vi "VI Erw. Konfig.vi"() -> ()   [LabVIEW 2020, in "Erweiterte Konfig.lvlib"]
uses:
  Seiten/Erweiterte Konfig/Erweiterte Konfig.lvlib
  Seiten/Erweiterte Konfig/PID-Parameter Anzeige.ctl
  Seiten/Erweiterte Konfig/PID-Parameter.ctl
  Visualisierungs Elemente/Zahlen-Eingabefeld.ctl
  Visualisierungs Elemente/Zahlen-Ausgabefeld.ctl
  Visualisierungs Elemente/Button.ctl
  Visualisierungs Elemente/Auswahlfeld.ctl
  Seiten/Erweiterte Konfig/Dichtheitstest Umfang.ctl
  Seiten/Erweiterte Konfig/Cluster LN2 normal.ctl
  Seiten/Erweiterte Konfig/Ventilanzeige.ctl
  Seiten/Erweiterte Konfig/Cluster Extern LN2.ctl
  Visualisierungs Elemente/String - Ausgabefeld.ctl
  Seiten/Erweiterte Konfig/Parameter Sensoren.ctl
  Seiten/Erweiterte Konfig/Aktionen Stickstoff Befuellung.ctl
  Seiten/Erweiterte Konfig/Aktionen Externe Stockstoff Befuellung.ctl
  Seiten/Erweiterte Konfig/FGV PID Aktionen.ctl
  Seiten/Log Konfig/Auswahlfeld aktiviert-deaktiviert.ctl
  Sprachverwaltung/FGV Aktion Tabelle zerlegen.ctl
  Passwortverwaltung/FGV Passwort Aktion.ctl
  Allgemein/Aktionen Daten am cRIO speichern.ctl
  Funktionstasten/Funktionstasten-Aktion.ctl
  Funktionstasten/Zustaende.ctl
  T90/T90 konfig.vi
  Seiten/Erweiterte Konfig/Parameter Druck Sensoren.vi
  Seiten/Erweiterte Konfig/PID-Parameter Druckregler einstellen v2.vi
  AK-Schnittstelle/Konfig AK.vi
  O2 Dichtheitstest/O2 main.vi
  Seiten/Erweiterte Konfig/Konfig CG-Check/VI CG-Check Konfig.vi
  Passwortverwaltung/Passwort.lvlib
  cRIO/PC/Kommunikation mit cRIO.lvlib
  Allgemein/allgemeine Sub-VIs.lvlib
  Funktionstasten/Funktionstasten.lvlib
  AK-Schnittstelle/AK-Schnittstelle.lvlib
  Seiten/Log Konfig/LogKonfig.lvlib
  T90/T90.lvlib
  Seiten/Erweiterte Konfig/Konfig CG-Check/CG-Check Konfig.lvlib
  O2 Dichtheitstest/O2 Dichtheitstest.lvlib
  Sprachverwaltung/Sprachverwaltung.lvlib
panel:
  in  "Aktion Externe Stickstoffbefüllung":T1
  in  "Aktion Stick":T2
  in  "O2 Dichtheitstest":T3 caption="Dichtheitstest"
  in  "Pumpendrehzahl":sgl=50.0 caption="Pumpendrehzahl:" min=50 max=100 format="%#_5g"
  in  "CG-Konfig":T3 caption="Dichtheitstest"
  out "Taupunkt":T4 caption="°C" format="%.1f"
  in  "Max Taupunkt":T5 caption="Offset Ausgang" format="%.1f"
  in  "Sensor Parameter":T3 caption="Status Digital IO"
  in  "Manueller Betrieb":bool
  in  "Gasringverdichter Speed":dbl(knob) scale=0.0..5.0
  out "Druck Umgebung:":T4 caption="mbar"
  in  "Offset Umgebung":T5 format="%#_5g"
  out "Rohwert Umgebung":T4 format="%.3f"
  out "Druck Ausgang:":T4 caption="mbar"
  in  "Offset Ausgang":T5 format="%#_5g"
  out "Rohwert Ausgang":T4 format="%.3f"
  in  "speichern":T3
  in  "T90":T3
  in  "Dichtheitstest":T3
  in  "Parameter Druckregler":T3
  in  "Status Digital IO":T3
  in  "Config AK":T3
  out "Klima Einschalten":string
  out "Klima":string
  in  "Schnell ab:":T5 caption="°C" format="%#_5g"
  in  "Lüfter langsam":T5 format="%#_5g"
  out "Rohwert Druck FT-IR":T4 format="%.3f"
  in  "Offset Druck FT-IR":T5 format="%#_5g"
  out "FT-IR Druck Ist":T4 format="%.3f"
  in  "Offset FT-IR":T5 format="%#_5g"
  out "Rohwert FT-IR":T4 format="%.3f"
  in  "Kalib.FT-IR":T5 format="%#_5g"
  in  "Registerkartenelement":T6(tab)
  in  "Dichtheitstest Umfang":T7 items=["FT-IR/PNS/HL to LeakValve", "FT-IR/PNS"]
  in  "Überwachung":T8 items=["Normaler Betrieb mit Überwachung", "Überwachung deaktiviert (TESTBETRIEB!!!!)"]
  in  "FT-IR Kühlung Max":T5 format="%.1f"
  out "FT-IR Kühlung Ist":T4 format="%.1f"
  in  "Dichtheitstest Zeit":T5 format="%#_5g"
  in  "Dichtheitstest Abfall":T5 format="%#_5g"
  in  "°C":T5 caption="Sollwert:" format="%.1f"
  in  "LN2 Cluster mit Ext":T9 {"Stickstoff Befüllzeit Ext" format="%#_5g"; "Befüllintervall" format="%#_5g"; "Stickstoff Befüllzeit" format="%#_5g"; "Befüllung Extern aktiv" items=["Deaktiviert", "Aktiviert"]; "Befüllung aktiv" items=["Deaktiviert", "Aktiviert"]}
  in  "LN2 normal":T12 {"Befüllung aktiv" items=["Deaktiviert", "Aktiviert"]; "Befüllintervall" format="%#_5g"; "Stickstoff Befüllzeit" format="%#_5g"}
  out "PMA unsichtbar schalten":bool
  out "Roh Druck Kalter Block":sgl caption="V" format="%.3f"
  out "Druck Kalter Block":sgl caption="bar" format="%.2f"
  out "Roh Durck FTIR IAG":sgl caption="V" format="%.3f"
  out "Roh Durck CG":sgl caption="V" format="%.3f"
  out "Roh Druck CG PMA":sgl caption="V" format="%.3f"
  out "Roh Durchfl.PMA":sgl caption="V" format="%.3f"
  out "Roh Durck Umgebung":sgl caption="V" format="%.3f"
  out "Roh Druck Ausgang":sgl caption="V" format="%.3f"
  out "Roh Durchfl.FTIR":sgl caption="V" format="%.3f"
  out "Druck FTIR IAG":sgl caption="atm" format="%.3f"
  out "Druck CG":sgl caption="bar" format="%.2f"
  out "Druck CG PMA":sgl caption="bar" format="%.2f"
  out "Druck Umgebung":sgl caption="mbar" format="%#.0f"
  out "Druck Ausgang":sgl caption="mbar" format="%#.0f"
  out "Durchfluss PMA":sgl caption="l/min" format="%.1f"
  out "Durchfluss FTIR":sgl caption="l/min" format="%.1f"
  in  "Parameter Sensoren":T13 {"Druck Kalter Block" format="%#_5g"; "Offset Druck FTIR IAG" format="%#_5g"; "Offset Druck CG" format="%#_5g"; "Offset Druck CG PMA" format="%#_5g"; "Offset Durchfl.PMA" format="%#_5g"; "Offset Druck Umgebung" format="%#_5g"; "Offset Druck Ausgang" format="%#_5g"; "Offset Durchfl.FTIR" format="%#_5g"; "Kal.Durchfl.PMA" format="%.3g"; "Kal.Durchfl.FTIR" format="%.3g"}
  in  "PID-Parameter Anzeige":T14 {"Heizung\nHeizleitungen"."max. OUT" format="%#_5g"; "Heizung\nHeizleitungen"."Regelzonengr." format="%#_5g"; "Heizung\nHeizleitungen"."D-Anteil" format="%#_5g"; "Heizung\nHeizleitungen"."I-Anteil" format="%#_5g"; "Heizung\nHeizleitungen"."P-Anteil" format="%.1f"; "Heizleitung\nExtern"."max. OUT" format="%#_5g"; "Heizleitung\nExtern"."Regelzonengr." format="%#_5g"; "Heizleitung\nExtern"."D-Anteil" format="%#_5g"; "Heizleitung\nExtern"."I-Anteil" format="%#_5g"; "Heizleitung\nExtern"."P-Anteil" format="%.1f"; "Heizung\nFB-Druckregler"."max. OUT" format="%#_5g"; "Heizung\nFB-Druckregler"."Regelzonengr." format="%#_5g"; "Heizung\nFB-Druckregler"."D-Anteil" format="%#_5g"; "Heizung\nFB-Druckregler"."I-Anteil" format="%#_5g"; "Heizung\nFB-Druckregler"."P-Anteil" format="%.1f"; "Heizung\nPumpe"."max. OUT" format="%#_5g"; "Heizung\nPumpe"."Regelzonengr." format="%#_5g"; "Heizung\nPumpe"."D-Anteil" format="%#_5g"; "Heizung\nPumpe"."I-Anteil" format="%#_5g"; "Heizung\nPumpe"."P-Anteil" format="%.1f"; "Heizung\nFilterblock"."max. OUT" format="%#_5g"; "Heizung\nFilterblock"."Regelzonengr." format="%#_5g"; "Heizung\nFilterblock"."D-Anteil" format="%#_5g"; "Heizung\nFilterblock"."I-Anteil" format="%#_5g"; "Heizung\nFilterblock"."P-Anteil" format="%.1f"}
  # "Erweiterte Konfig"
  # "°C"
  # "%"
  # "Taupunktsensor:"
  # "Istwert:"
  # "°C"
  # "Max. Wert:"
  # "Istwert:"
  # "Umgebungsdruck:"
  # "Offset:"
  # "mbar"
  # "Rohwert:"
  # "V"
  # "Istwert:"
  # "Druck Ausgang:"
  # "Offset:"
  # "mbar"
  # "Rohwert:"
  # "V"
  # "Istwert:"
  # "Druck FT-IR IAG:"
  # "atm"
  # "Offset:"
  # "atm"
  # "Rohwert:"
  # "V"
  # "Durchfluss FT-IR:"
  # "Kalibrierwert:"
  # "Offset:"
  # "Rohwert:"
  # "V"
  # "Dichtheitstest:"
  # "max. Druckanstieg:"
  # "mbar"
  # "Kühlung FT-IR:"
  # "Max. Wert:"
  # "°C"
  # "Überwachung von Grundbedingnungen:"
  # "Istwert:"
  # "°C"
  # "Prüfzeit:"
  # "sec"
  # "Parameter interne Flüssig-Stickstoff-Nachfüllung"
  # "Parameter externe Flüssig-Stickstoff-Nachfüllung"
  # "PA"
  # "3"
  # "Externer\nDewar 50l"
  # "Dewar 4l"
  # "FT-IR"
  # "Zeitdauer letzter Füllvorgang:"
  # "sec"
  # "Fülldauer wenn Sensor erkannt:"
  # "sec"
  # "Befüllintervall:"
  # "Stunden"
  # "Zeitdauer letzter Füllvorgang:"
  # "sec"
  # "Fülldauer wenn Sensor erkannt:"
  # "sec"
  # "N2"
  # "5"
  # "CA"
  # "3"
  # "LS"
  # "-16B1"
  # "LS"
  # "-17B2"
  # "LS"
  # "-16B2"
  # "LS"
  # "-17B3"
  # "PR"
  # "0,2bar"
  # "Parameter interne Flüssig-Stickstoff-Nachfüllung"
  # "Zustand Befüllsystem:"
  # "Befüllintervall:"
  # "Stunden"
  # "Zeitstempel - letzter Füllvorgang:"
  # "Zeitdauer letzter Füllvorgang:"
  # "sec"
  # "Fülldauer wenn Sensor erkannt:"
  # "sec"
  # "Zeitstempel - vorletzter Füllvorgang:"
  # "Dewar 4l"
  # "FT-IR"
  # "N2"
  # "5"
  # "CA"
  # "3"
  # "LS"
  # "-16B1"
  # "LS"
  # "-16B2"
  # "Sensor"
  # "Istwert"
  # "Kalibrierwert"
  # "Offset"
  # "Rohwert"
  # "Durchfluss FT-IR:"
  # "Druck Ausgang:"
  # "Ambient Pressure:"
  # "Druck Calgas:"
  # "Druck FT-IR IAG:"
  # "Fluss PMA:"
  # "Druck CG PMA:"
  # "Druck Kalter Block:"
  # "PID -Parameter:"
  # "Verstärkung KR:"
  # "Nachstellzeit TN:"
  # "Vorhaltezeit TD:"
  # "Regelzonengrenze:"
  # "max. Ausgang:"
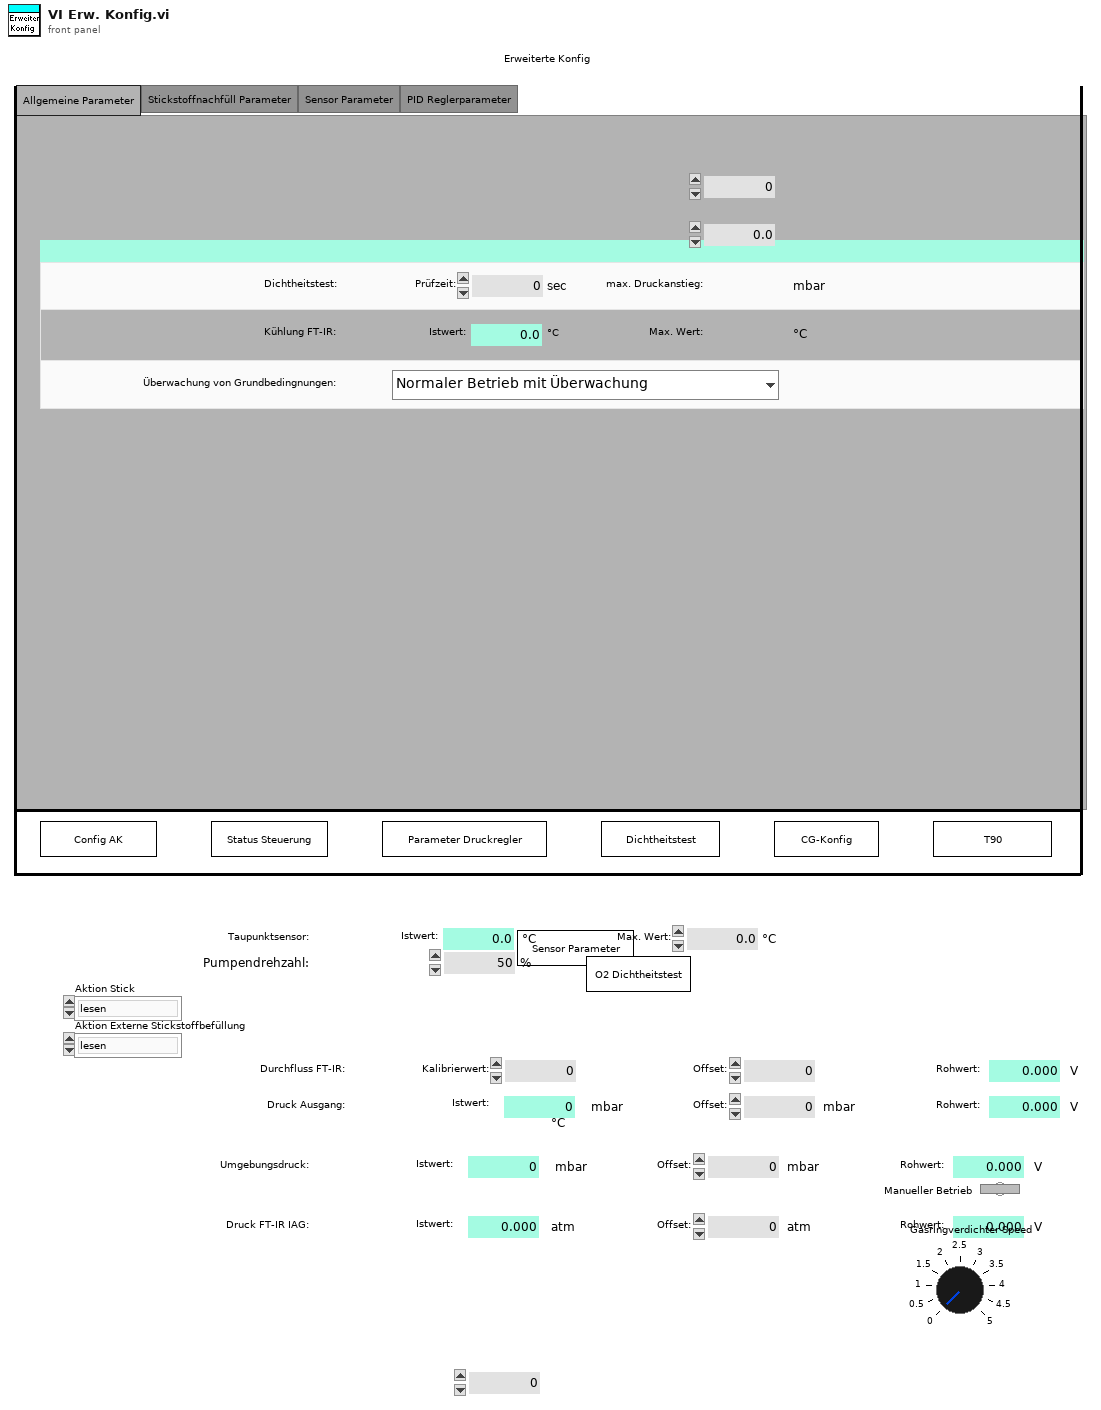
[diagram p1: front panel]
types:
  T1 = typedef "Erweiterte Konfig.lvlib/Aktionen Externe Stockstoff Befuellung.ctl" = enum16{"lesen", "Befüllen vorbereiten", "Befüllen", "Befüllen beenden", "Warten", "deaktiviert", "initialisieren"}
  T2 = typedef "Erweiterte Konfig.lvlib/Aktionen Stickstoff Befuellung.ctl" = enum16{"lesen", "Befüllen vorbereiten", "Befüllen", "Befüllen beenden", "Warten", "deaktiviert", "initialisieren"}
  T3 = typedef "Button.ctl" = bool
  T4 = typedef "Zahlen-Ausgabefeld.ctl" = sgl
  T5 = typedef "Zahlen-Eingabefeld.ctl" = sgl
  T6 = enum32{"General Parameters", "Liquid Nitrogen Parameters", "Sensor Parameter", "PID Regulate Parameters"}
  T7 = typedef "Erweiterte Konfig.lvlib/Dichtheitstest Umfang.ctl" = u16
  T8 = typedef "Auswahlfeld.ctl" = u16
  T9 = typedef "Erweiterte Konfig.lvlib/Cluster Extern LN2.ctl" = cluster{"Befüllung aktiv":u16, "Zeitstempel":timestamp, "Zeitstempel 2":timestamp, "Status LN2 Befüllung":T10, "Befüllintervall":T5, "Zeit Füllvorgang":T4, "Stickstoff Befüllzeit":T5, "Befüllung Extern aktiv":u16, "Zeitstempel 1 Ext":timestamp, "Zeitstempel 2 Ext":timestamp, "Status LN2 Befüllung Ext.":T10, "Zeit Füllvorgang Ext":T4, "Stickstoff Befüllzeit Ext":T5, "LS -17B3":bool, "LS -16B2":bool, "LS -17B2":bool, "-22Y3 ":T11, "-22Y1":T11, "LS -16B1":bool, "-16B7":bool, "-22Y2":T11}
  T10 = typedef "String - Ausgabefeld.ctl" = string
  T11 = typedef "Erweiterte Konfig.lvlib/Ventilanzeige.ctl" = bool
  T12 = typedef "Erweiterte Konfig.lvlib/Cluster LN2 normal.ctl" = cluster{"Zeitstempel":timestamp, "Zeitstempel 2":timestamp, "Zeit Füllvorgang":T4, "Stickstoff Befüllzeit":T5, "Befüllintervall":T5, "Befüllung aktiv":u16, "-22Y1":T11, "-22Y2":T11, "LS -16B1":bool, "LS -16B2":bool}
  T13 = typedef "Erweiterte Konfig.lvlib/Parameter Sensoren.ctl" = cluster{"Kal.Durchfl.FTIR":sgl, "Kal.Durchfl.PMA":sgl, "Offset Durchfl.FTIR":sgl, "Offset Druck Ausgang":sgl, "Offset Druck Umgebung":sgl, "Offset Durchfl.PMA":sgl, "Offset Druck CG PMA":sgl, "Offset Druck CG":sgl, "Offset Druck FTIR IAG":sgl, "Druck Kalter Block":sgl}
  T14 = typedef "Erweiterte Konfig.lvlib/PID-Parameter Anzeige.ctl" = cluster{"Heizung\nFilterblock":T15, "Heizung\nPumpe":T15, "Heizung\nHeizleitungen":T15, "Heizleitung\nExtern":T15, "Heizung\nFB-Druckregler":T15}
  T15 = typedef "Erweiterte Konfig.lvlib/PID-Parameter.ctl" = cluster{"P-Anteil":T5, "I-Anteil":T5, "D-Anteil":T5, "Regelzonengr.":T5, "max. OUT":T5}
  T16 = typedef "Sprachverwaltung.lvlib/FGV Aktion Tabelle zerlegen.ctl" = enum16{"laden", "vereinzeln", "speichern"}
  T17 = enum8{"Enabled", "Disabled", "Disabled and Grayed Out"}
  T18 = typedef "Erweiterte Konfig.lvlib/FGV PID Aktionen.ctl" = enum16{"Lesen", "Schreiben PID", "Schreiben Sonstige", "Dichtheitstest", "Aktionen Dicht.", "Parameter Sensor"}
  T19 = typedef "LogKonfig.lvlib/Auswahlfeld aktiviert-deaktiviert.ctl" = u16
  T20 = typedef "Erweiterte Konfig.lvlib/Sonstige Parameter.ctl" = cluster{"Lüfter langsam":sgl, "Lüfter schnell":sgl, "FT-IR Kühlung Soll":sgl, "FT-IR Kühlung Max":sgl, "Überwachung":T8, "Befüllung aktiv":T19, "Stickstoff Befüllzeit":sgl, "Befüllintervall":sgl, "Kalibrierwert FT-IR":sgl, "Offset Ausgang":sgl, "Offset FT-IR":sgl, "Offset Druck FT-IR":sgl, "Dichtheitstest Zeit":sgl, "Dichtheitstest Abfall":sgl, "Dichtheitstest Umfang":T7, "Offset Umgebung":sgl, "Max Taupunkt":sgl, "Pumpendrehzahl":sgl, "ext. Befüllung":T19, "Ext. Stickstoff Befüllzeit":sgl}
  T21 = typedef "Passwort.lvlib/FGV Passwort Aktion.ctl" = enum16{"prüfen", "setzen", "Initialisieren", "PW speichern", "lesen", "PW Änderung"}
  T22 = typedef "allgemeine Sub-VIs.lvlib/Aktionen Daten am cRIO speichern.ctl" = enum16{"lesen", "speichern setzen", "speichern reset", "gespeichert"}
  T23 = typedef "Funktionstasten.lvlib/Zustaende.ctl" = enum16{"Standby", "Pause", "Eco", "Messen", "Kalibrieren", "Spülen Filter", "Spülen Leitung", "Umgebungsluft", "0-Gas", "Cal-Gas", "CG zu PNS", "-------------", "Init 1", "Init 2", "Init 3", "Init 4", "Messen vorbereiten", "Messen durchführen", "Exit"}
  T24 = typedef "Funktionstasten.lvlib/Funktionstasten-Aktion.ctl" = enum16{"Initialisieren", "Zustand setzen", "Taste gedrückt", "Fehler speichern", "Lesen", "Manuell", "Remote", "Bitparallel", "Samplepoint", "Zeit Prüfen", "reset Umschalten"}
  T25 = typedef "Verwaltung - cRIO.lvlib/Digital Eingaenge 0-15.ctl" = cluster{"I0: N2 Nachf. FT-IR voll":bool, "I1: N2 Nachf. Vorrat leer":bool, "I2: (Klimaanlage eingeschaltet)":bool, "I3: (Klimaanlage Störung)":bool, "I4: Trigger Eingang (Messdaten sp.)":bool, "I5: Reserve":bool, "I6: Reserve":bool, "I7: Reserve":bool, "I8: Druckschalter Versorgung ok":bool, "I9: Reserve":bool, "I10: Reserve":bool, "I11: Reserve":bool, "I12: Drucksch. N2 Versorgung":bool, "I13: Reserve":bool, "I14: Drucksch. N2 Optikbox":bool, "I15: (Füllstand Kondensatbehälter)":bool}
  T26 = typedef "Verwaltung - cRIO.lvlib/Digital Ausgaenge 0-31.ctl" = cluster{"O0: Druckluft Versorgung":bool, "O1: CG 1 (FB Eingang 1)":bool, "O2: CG 2 (Kühlung FT-IR EIN)":bool, "O3: CG 3 (FB Bypass)":bool, "O4: CG 4 (FB CalGas)":bool, "O5: CG 5 (FB spülen/UL)":bool, "O6: CG 6 (FB zum FT-IR)":bool, "O7: CG 7 (FB zum FID)":bool, "O8: CG 8 (FB Reserve)":bool, "O9: (FB Reserve)":bool, "O10: (FB Umgebungsluft FID)":bool, "O11: (FB zum Gaskühler)":bool, "O12: FB Stickstoff zu FT-IR":bool, "O13: Optikbox FT-IR spülen":bool, "O14: (Purifier deaktivieren)":bool, "O15: (Umschaltung Purifier/Stickstoff)":bool, "O16: N2 Einblasung":bool, "O17: LSP LN2 Nachfüllung":bool, "O18: (Reserve)":bool, "O19: (Pumpe Eingang1)":bool, "O20: (Pumpe Eingang2)":bool, "O21: (Pumpe Spülen1)":bool, "O22: (Pumpe Spülen2)":bool, "O23: (Reserve)":bool, "O24: CalGas 1":bool, "O25: CalGas 2":bool, "O26: CG 3-8 (CalGas 3)":bool, "O27: Stickstoff aufschalten":bool, "O28: CG zu PNS":bool, "O29: FTIR Standby Spülung":bool, "O30: CG zu Entnahme(T90)":bool, "O31: (Purifier regenerieren)":bool}
  T27 = typedef "Verwaltung - cRIO.lvlib/Digital Ausgaenge 32-63.ctl" = cluster{"O32: Messgaspumpe EIN":bool, "O33: (Umgebungsluftpumpe)":bool, "O34: (Kondensatpumpe GK)":bool, "O35: Klima/Lüfter EIN":bool, "O36: Versorgung Heizungen":bool, "O37: Versorgung Heizungen":bool, "O38: (Gaskühler EIN (Freigabe))":bool, "O39: Störung FAS LP":bool, "O40: (Heizung Filterblock)":bool, "O41: Heizung HL zu FT-IR":bool, "O42: Heizung HL Extern SP1":bool, "O43: Heizung HL Extern SP2":bool, "O44: Heizung Reserve":bool, "O45: Heizung Reserve":bool, "O46: Statusbeleuchtung grün":bool, "O47: Statusbeleuchtung rot":bool}
  T28 = typedef "Verwaltung - cRIO.lvlib/Analog Eingaenge.ctl" = cluster{"AI0: Durchfluss FT-IR":sgl, "AI1: Druck Ausgang":sgl, "AI2: Umgebungsdruck":sgl, "AI3: Druck FT-IR":sgl, "AI4: Druck CalGas":sgl, "AI5: Reserve":sgl, "AI6: Reserve":sgl, "AI7: Reserve":sgl, "Rohwert Durchfluss FT-IR":sgl, "Rohwert Druck Ausgang":sgl, "Rohwert Umgebungsdruck":sgl, "Rohwert Druck FT-IR":sgl, "Rohwert Druck CalGas":sgl, "Rohwert AI5":sgl, "Rohwert AI6":sgl, "Rohwert AI7":sgl, "Rohwert Diffdruck mbar FTIR":sgl}
  T29 = typedef "Verwaltung - cRIO.lvlib/TC Eingaenge.ctl" = cluster{"TC0: Reserve":sgl, "TC1: HL zu FT-IR":sgl, "TC2: HL Extern SP1":sgl, "TC3: HL Extern SP2":sgl, "TC4: Reserve":sgl, "TC5: Reserve":sgl, "TC6: Reserve":sgl, "TC7: Reserve":sgl, "TC8: FT-IR":sgl, "TC9: Reserve":sgl, "TC10: Schaltschrank":sgl, "TC11: Umgebung":sgl}
  T30 = cluster{"Lüfter langsam":T5, "Schnell ab:":T5, "°C":T5, "FT-IR Kühlung Max":T5, "Überwachung":T8, "Befüllung aktiv":u16, "Stickstoff Befüllzeit":T5, "Befüllintervall":T5, "Kalib.FT-IR":T5, "Offset Ausgang":T5, "Offset FT-IR":T5, "Offset Druck FT-IR":T5, "Dichtheitstest Zeit":T5, "Dichtheitstest Abfall":T5, "Dichtheitstest Umfang":T7, "Offset Umgebung":T5, "Max Taupunkt":T5, "Pumpendrehzahl":sgl, "Befüllung Extern aktiv":u16, "Stickstoff Befüllzeit Ext":T5}
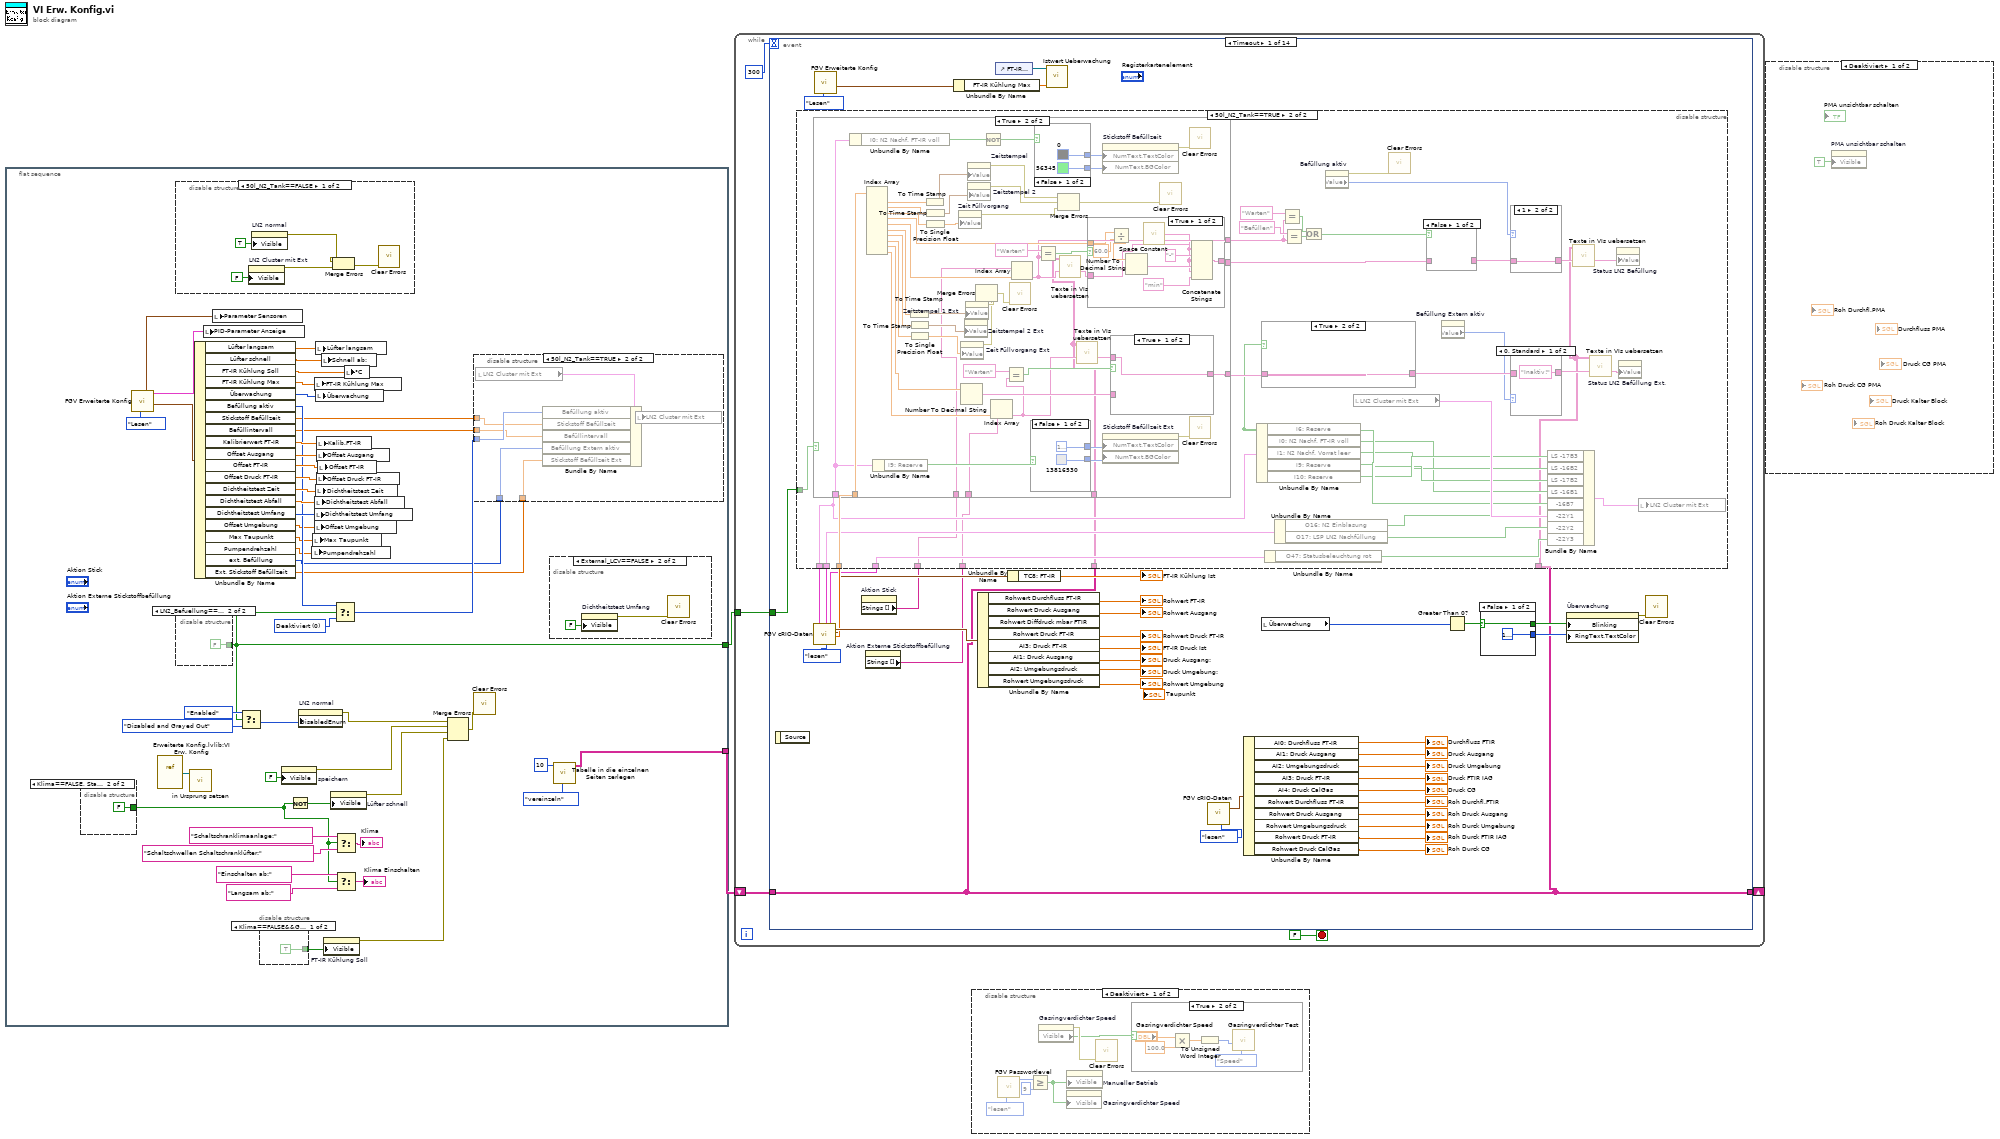
[diagram p0: block diagram]
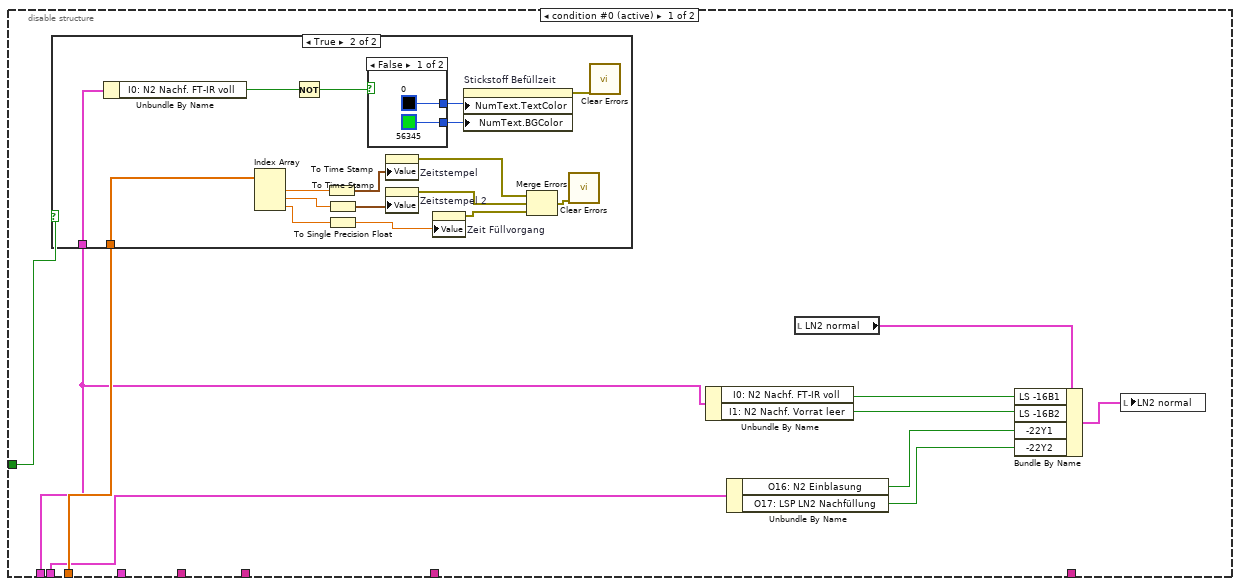
[diagram p5: hidden frame]
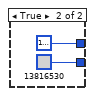
[diagram p7: hidden frame]
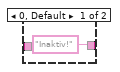
[diagram p9: hidden frame]
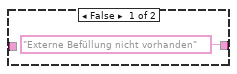
[diagram p10: hidden frame]
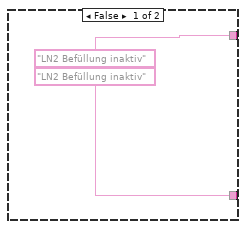
[diagram p12: hidden frame]
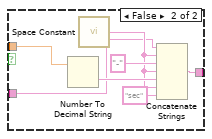
[diagram p13: hidden frame]
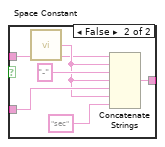
[diagram p14: hidden frame]
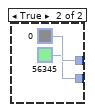
[diagram p15: hidden frame]
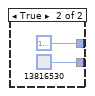
[diagram p16: hidden frame]
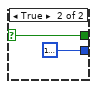
[diagram p17: hidden frame]
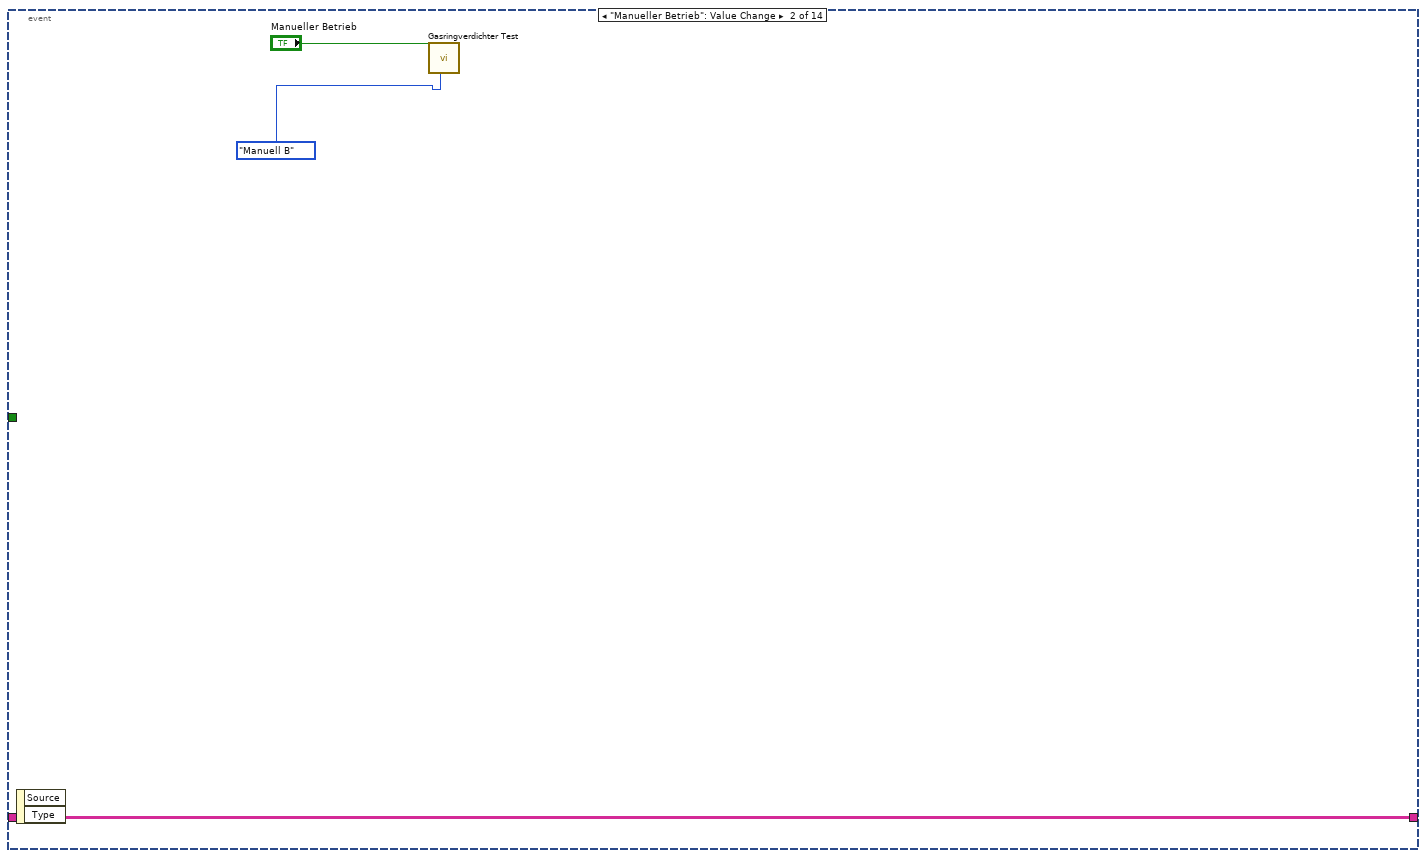
[diagram p18: hidden frame]
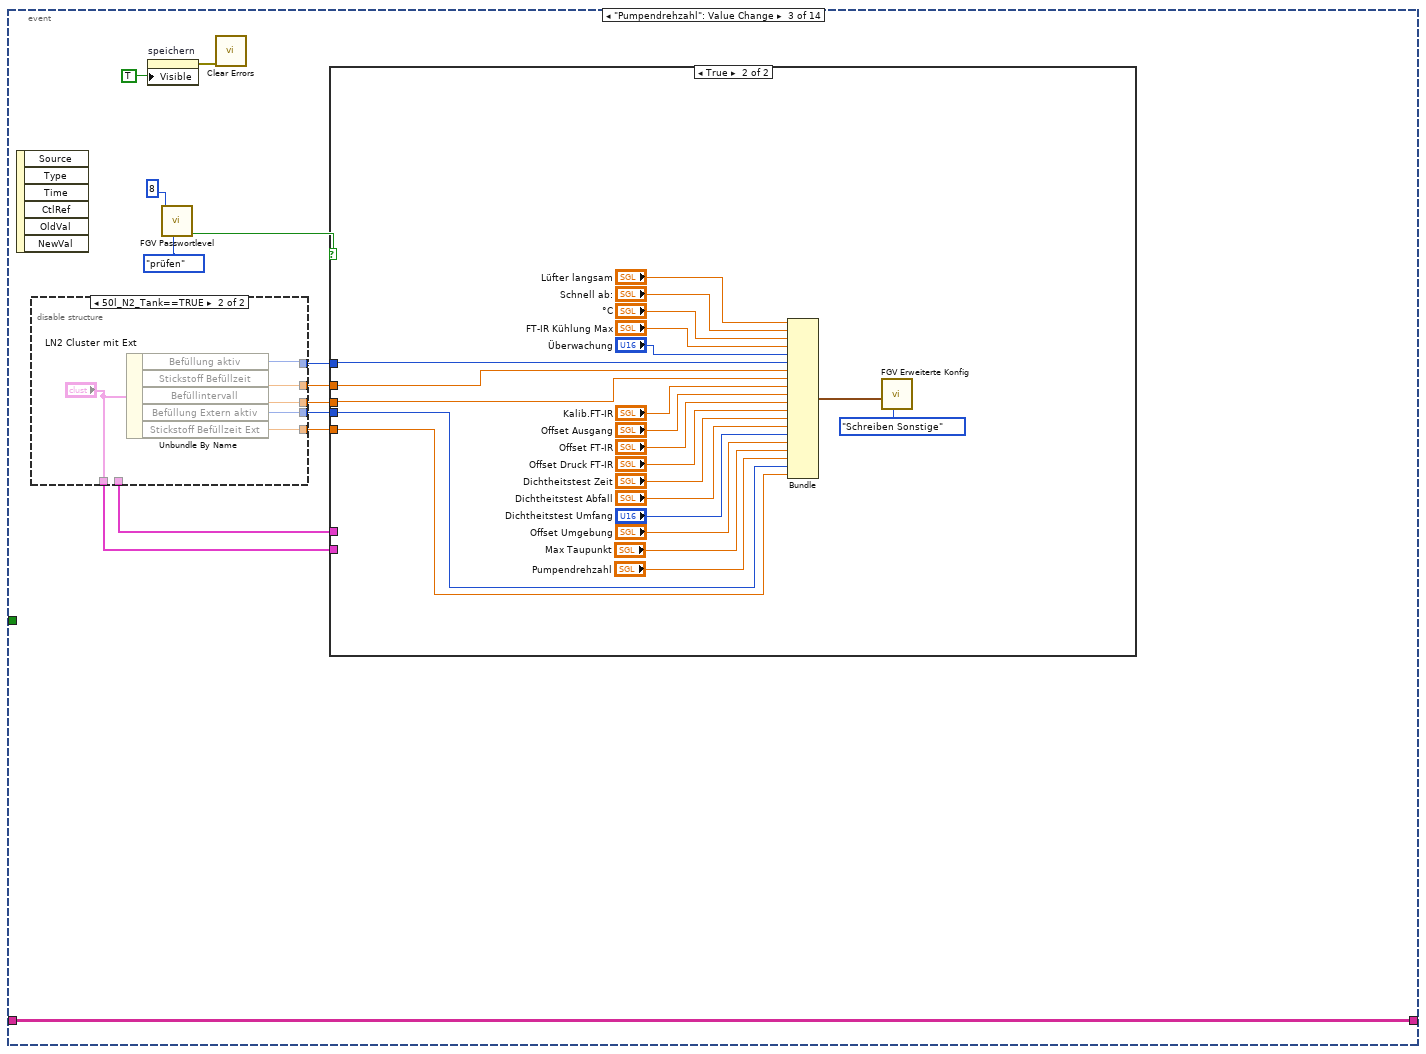
[diagram p19: hidden frame]
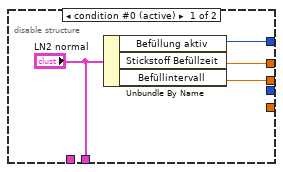
[diagram p20: hidden frame]
diagram:
  n1 = flat-sequence {
    tunnel: [w30] -> w2
    tunnel: [w4] -> w1
    frame #0 {
      w31 = T19 0 items=["Deaktiviert", "Aktiviert"] ("f")
      n2 = disable-structure shown="Klima==FALSE, Standard" {
        disable-tunnel: [TRUE ("Klimaanlage ?") FALSE ("Klimaanlage ?")] -> w19
        frame condition #0 {
        }
        frame condition #1 (active) {
        }
      }
      n3 = call "FGV Erweiterte Konfig.vi"("Aktion"=FGV_PID_Aktionen."Lesen") -> ("Sonstige"=w49:T20, "PID-Parameter Anzeige"=w50:T14, "Parameter Sensoren"=w3:T13)  [unwired: 5 in, 3 out]
      n4 = vi-ref "Erweiterte Konfig.lvlib:VI Erw. Konfig.vi"() -> (w34:refnum<vi>)
      n5 = disable-structure shown="50l_N2_Tank==FALSE" {
        frame condition #0 (active) {
          n6 = property on="LN2 Cluster mit Ext" class="Cluster (strikt)"("Visible"=FALSE ("Sichtbar")) -> (error out=w73:errorcluster)  [unwired: 2 in, 1 out]
          n7 = property on="LN2 normal" class="Cluster (strikt)"("Visible"=TRUE ("Sichtbar")) -> (error out=w74:errorcluster)  [unwired: 2 in, 1 out]
          n8 = Merge Errors(w74, w73) -> (w72:errorcluster)
          n9 = call <vilib>:"Clear Errors.vi"("error in (no error)"=w72) -> ()  [unwired: 5 in, 2 out]
        }
        frame condition #1 {
          n10 = property on="LN2 Cluster mit Ext" class="Cluster (strikt)"("Visible"=TRUE ("Sichtbar")) -> (error out=w76:errorcluster)  [unwired: 2 in, 1 out]
          n11 = property on="LN2 normal" class="Cluster (strikt)"("Visible"=FALSE ("Sichtbar")) -> (error out=w77:errorcluster)  [unwired: 2 in, 1 out]
          n12 = Merge Errors(w77, w76) -> (w75:errorcluster)
          n13 = call <vilib>:"Clear Errors.vi"("error in (no error)"=w75) -> ()  [unwired: 5 in, 2 out]
        }
      }
      n14 = disable-structure shown="LN2_Befuellung==FALSE" {
        disable-tunnel: [TRUE ("LN2 Befüllung") FALSE ("LN2 Befüllung")] -> w30
        frame condition #0 (active) {
        }
        frame condition #1 {
        }
      }
      n15 = call "in Ursprung setzen.vi"("VI Referenz"=w34) -> ()  [unwired: 10 in, 1 out]
      n16 = Unbundle By Name(w49) -> ("Lüfter langsam"=w48:sgl, "Lüfter schnell"=w47:sgl, "FT-IR Kühlung Soll"=w46:sgl, "FT-IR Kühlung Max"=w45:sgl, "Überwachung"=w44:T8, "Befüllung aktiv"=w32:T19, "Stickstoff Befüllzeit"=w10:sgl, "Befüllintervall"=w9:sgl, "Kalibrierwert FT-IR"=w43:sgl, "Offset Ausgang"=w42:sgl, "Offset FT-IR"=w41:sgl, "Offset Druck FT-IR"=w40:sgl, "Dichtheitstest Zeit"=w39:sgl, "Dichtheitstest Abfall"=w38:sgl, "Dichtheitstest Umfang"=w37:T7, "Offset Umgebung"=w18:sgl, "Max Taupunkt"=w17:sgl, "Pumpendrehzahl"=w16:sgl, "ext. Befüllung"=w8:T19, "Ext. Stickstoff Befüllzeit"=w7:sgl)
      n17 = local write "PID-Parameter Anzeige"(w50) -> ()
      n18 = local write "Parameter Sensoren"(w3) -> ()
      n19 = Select(t=T17."Enabled" ("Deaktiviert"), s=w30, f=T17."Disabled and Grayed Out" ("Deaktiviert")) -> (s? t:f=w13:T17)
      n20 = disable-structure shown="Klima==FALSE&&Gehaeuseluefter==FALSE, Standard" {
        disable-tunnel: [TRUE FALSE] -> w14
        frame condition #0 {
        }
        frame condition #1 (active) {
        }
      }
      n21 = property on="speichern" class="Bool."("Visible"=FALSE ("Sichtbar")) -> (error out=w29:errorcluster)  [unwired: 2 in, 1 out]
      n22 = Not(x=w19) -> (.not. x?=w20:bool)
      n23 = property on="LN2 normal" class="Cluster (strikt)"("DisabledEnum"=w13) -> (error out=w12:errorcluster)  [unwired: 2 in, 1 out]
      n24 = local write "Pumpendrehzahl"(w16) -> ()
      n25 = local write "Max Taupunkt"(w17) -> ()
      n26 = local write "Dichtheitstest Umfang"(w37) -> ()
      n27 = local write "Offset Umgebung"(w18) -> ()
      n28 = local write "FT-IR Kühlung Max"(w45) -> ()
      n29 = local write "Dichtheitstest Abfall"(w38) -> ()
      n30 = local write "Lüfter langsam"(w48) -> ()
      n31 = local write "Überwachung"(w44) -> ()
      n32 = local write "Dichtheitstest Zeit"(w39) -> ()
      n33 = local write "Offset Ausgang"(w42) -> ()
      n34 = local write "Offset Druck FT-IR"(w40) -> ()
      n35 = local write "Kalib.FT-IR"(w43) -> ()
      n36 = local write "Offset FT-IR"(w41) -> ()
      n37 = local write "Schnell ab:"(w47) -> ()
      n38 = property on="FT-IR Kühlung Soll" class="DigWert (strikt)"("Visible"=w14) -> (error out=w15:errorcluster)  [unwired: 2 in, 1 out]
      n39 = property on="Lüfter schnell" class="DigWert (strikt)"("Visible"=w20) -> (error out=w21:errorcluster)  [unwired: 2 in, 1 out]
      n40 = Select(t=w32, s=w30, f=w31) -> (s? t:f=w11:T19)
      n41 = Select(t="Schaltschranklimaanlage:", s=w19, f="Schaltschwellen Schaltschranklüfter:") -> (s? t:f=→"Klima":string)
      n42 = Select(t="Einschalten ab:", s=w19, f="Langsam ab:") -> (s? t:f=→"Klima Einschalten":string)
      n43 = local write "°C"(w46) -> ()
      n44 = Merge Errors(w12, w29, w21, w15) -> (w28:errorcluster)
      n45 = disable-structure shown="50l_N2_Tank==TRUE" {
        disable-tunnel: w11 -> [w61 w67]
        disable-tunnel: w10 -> [w60 w66]
        disable-tunnel: w9 -> [w59 w65]
        disable-tunnel: w8 -> [_ w64]
        disable-tunnel: w7 -> [_ w63]
        frame condition #0 (active) {
          n46 = local read "LN2 normal"() -> (w62:T12)
          n47 = Bundle By Name(cluster=w62, "Stickstoff Befüllzeit"=w60, "Befüllintervall"=w59, "Befüllung aktiv"=w61) -> (w58:T12)
          n48 = local write "LN2 normal"(w58) -> ()
        }
        frame condition #1 {
          n49 = local read "LN2 Cluster mit Ext"() -> (w69:T9)
          n50 = Bundle By Name(cluster=w69, "Befüllung aktiv"=w67, "Stickstoff Befüllzeit"=w66, "Befüllintervall"=w65, "Befüllung Extern aktiv"=w64, "Stickstoff Befüllzeit Ext"=w63) -> (w68:T9)
          n51 = local write "LN2 Cluster mit Ext"(w68) -> ()
        }
      }
      n52 = call <vilib>:"Clear Errors.vi"("error in (no error)"=w28) -> ()  [unwired: 5 in, 2 out]
      n53 = disable-structure shown="External_LCV==FALSE" {
        frame condition #0 {
          n54 = property on="Dichtheitstest Umfang" class="Ring (strikt)"("Visible"=TRUE ("Sichtbar")) -> (error out=w52:errorcluster)  [unwired: 2 in, 1 out]
          n55 = call <vilib>:"Clear Errors.vi"("error in (no error)"=w52) -> ()  [unwired: 5 in, 2 out]
        }
        frame condition #1 (active) {
          n56 = property on="Dichtheitstest Umfang" class="Ring (strikt)"("Visible"=FALSE ("Sichtbar")) -> (error out=w54:errorcluster)  [unwired: 2 in, 1 out]
          n57 = call <vilib>:"Clear Errors.vi"("error in (no error)"=w54) -> ()  [unwired: 5 in, 2 out]
        }
      }
      n58 = call "Tabelle in die einzelnen Seiten zerlegen.vi"("Aktion"=FGV_Aktion_Tabelle_zerlegen."vereinzeln", "Index (Seite)"=10) -> ("Sprachliste"=w4:string[][])  [unwired: 7 in, 2 out]
    }
  }
  n59 = while {
    tunnel: w2 -> [w86]
    shift-right: [w84] -> _
    shift-left: w1 -> [w85]
    stop <- FALSE stop-if-true
    n60 = event shown="[0] Timeout" {
      selector: _ -> [_ _ _ _ _ _ _ _ _ _ _ _ _ _]
      dyn-events: _ -> [_ _ _ _ _ _ _ _ _ _ _ _ _ _]
      timeout: 300 -> [_ _ _ _ _ _ _ _ _ _ _ _ _ _]
      tunnel: w86 -> [w113 _ _ _ _ _ _ _ _ _ _ _ _ _]
      tunnel: w85 -> [w101 w289 w292 w368 w370 w372 w377 w388 w393 w398 w400 w406 w408 w417]
      tunnel: [w101 w289 w292 w368 w370 w372 w377 w388 w393 w398 w400 w406 w408 w417] -> w84
      event Timeout {
        n61 = event-data() -> ()  [unwired: 2 out]
        n62 = call "FGV cRIO-Daten.vi"("Aktion"=enum16{"lesen", "schreiben"}."lesen") -> ("DI"=w114:T25, "DO 0-31"=w105:T26, "DO 32-63"=w104:T27, "Analog Input"=w125:T28, "TC Eingänge"=w108:T29, "Stickstoff Befüllung"=w115:dbl[])  [unwired: 9 in, 4 out]
        n63 = call "FGV Erweiterte Konfig.vi"("Aktion"=FGV_PID_Aktionen."Lesen") -> ("Sonstige"=w123:T20)  [unwired: 5 in, 5 out]
        n64 = property on="Aktion Stick" class="Enum (strikt)"() -> ("Strings []"=w103:string[])  [unwired: 2 in, 2 out]
        n65 = property on="Aktion Externe Stickstoffbefüllung" class="Enum (strikt)"() -> ("Strings []"=w102:string[])  [unwired: 2 in, 2 out]
        n66 = disable-structure shown="50l_N2_Tank==TRUE" {
          disable-tunnel: w115 -> [w138 w195]
          disable-tunnel: w114 -> [w135 w181]
          disable-tunnel: w113 -> [w137 w194]
          disable-tunnel: w105 -> [w136 w173]
          disable-tunnel: w104 -> [_ w170]
          disable-tunnel: w103 -> [_ w167]
          disable-tunnel: w102 -> [_ w166]
          disable-tunnel: w101 -> [_ w163]
          disable-tunnel: w101 -> [_ w162]
          frame condition #0 (active) {
            n67 = case shown="True" w137 {
              tunnel: w138 -> [_ w152]
              tunnel: w135 -> [_ w151]
              frame False {
              }
              frame True {
                n68 = Unbundle By Name(w151) -> ("I0: N2 Nachf. FT-IR voll"=w150:bool)
                n69 = Index Array(array=w152) -> (element #1=w153:dbl, element #2=w154:dbl, element #3=w155:dbl)  [unwired: 3 in]
                n70 = Not(x=w150) -> (.not. x?=w149:bool)
                n71 = To Time Stamp(1:w153) -> (0:w146:timestamp)
                n72 = To Time Stamp(1:w154) -> (0:w143:timestamp)
                n73 = To Single Precision Float(number=w155) -> (single precision float=w141:sgl)
                n74 = case shown="False" w149 {
                  tunnel: [u32 0 u32 16777222] -> w139
                  tunnel: [u32 56345 u32 13816530] -> w148
                  frame False {
                  }
                  frame True {
                  }
                }
                n75 = property on="Zeitstempel" class="AbsZeit (strikt)"("Value"=w146) -> (error out=w144:errorcluster)  [unwired: 2 in, 1 out]
                n76 = property on="Zeitstempel 2" class="AbsZeit (strikt)"("Value"=w143) -> (error out=w142:errorcluster)  [unwired: 2 in, 1 out]
                n77 = property on="Zeit Füllvorgang" class="DigWert (strikt)"("Value"=w141) -> (error out=w140:errorcluster)  [unwired: 2 in, 1 out]
                n78 = property on="Stickstoff Befüllzeit" class="DigWert (strikt)"("NumText.TextColor"=w139, "NumText.BGColor"=w148) -> (error out=w147:errorcluster)  [unwired: 2 in, 1 out]
                n79 = Merge Errors(w144, w142, w140) -> (w145:errorcluster)
                n80 = call <vilib>:"Clear Errors.vi"("error in (no error)"=w145) -> ()  [unwired: 5 in, 2 out]
                n81 = call <vilib>:"Clear Errors.vi"("error in (no error)"=w147) -> ()  [unwired: 5 in, 2 out]
              }
            }
            n82 = Unbundle By Name(w135) -> ("I0: N2 Nachf. FT-IR voll"=w132:bool, "I1: N2 Nachf. Vorrat leer"=w131:bool)
            n83 = Unbundle By Name(w136) -> ("O16: N2 Einblasung"=w130:bool, "O17: LSP LN2 Nachfüllung"=w129:bool)
            n84 = local read "LN2 normal"() -> (w134:T12)
            n85 = Bundle By Name(cluster=w134, "LS -16B1"=w132, "LS -16B2"=w131, "-22Y1"=w130, "-22Y2"=w129) -> (w133:T12)
            n86 = local write "LN2 normal"(w133) -> ()
          }
          frame condition #1 {
            n87 = case shown="True" w194 {
              tunnel: w195 -> [_ w248]
              tunnel: w181 -> [_ w244]
              tunnel: ["LN2 Befüllung inaktiv" w233] -> w185
              tunnel: ["LN2 Befüllung inaktiv" w232] -> w184
              tunnel: [_ w207] -> w186
              tunnel: w167 -> [_ w216]
              tunnel: w166 -> [_ w215]
              tunnel: w162 -> [_ w205]
              frame False {
              }
              frame True {
                n88 = Unbundle By Name(w244) -> ("I0: N2 Nachf. FT-IR voll"=w246:bool)
                n89 = Index Array(array=w248) -> (element #1=w249:dbl, element #2=w250:dbl, element #3=w251:dbl, element #4=w236:dbl, element #5=w235:dbl, element #6=w239:dbl, element #7=w238:dbl, element #8=w237:dbl, element #9=w234:dbl, element #10=w217:dbl)  [unwired: 10 in]
                n90 = Unbundle By Name(w244) -> ("I9: Reserve"=w240:bool)
                n91 = To Time Stamp(1:w239) -> (0:w223:timestamp)
                n92 = To Time Stamp(1:w238) -> (0:w222:timestamp)
                n93 = To Single Precision Float(number=w237) -> (single precision float=w221:sgl)
                n94 = To Time Stamp(1:w249) -> (0:w230:timestamp)
                n95 = To Time Stamp(1:w250) -> (0:w229:timestamp)
                n96 = To Single Precision Float(number=w251) -> (single precision float=w228:sgl)
                n97 = property on="Zeit Füllvorgang" class="DigWert (strikt)"("Value"=w228) -> (error out=w225:errorcluster)  [unwired: 2 in, 1 out]
                n98 = property on="Zeit Füllvorgang Ext" class="DigWert (strikt)"("Value"=w221) -> (error out=w218:errorcluster)  [unwired: 2 in, 1 out]
                n99 = Number To Decimal String(number=w234) -> (decimal integer string=w231:string)  [unwired: 1 in]
                n100 = property on="Zeitstempel 2 Ext" class="AbsZeit (strikt)"("Value"=w222) -> (error out=w219:errorcluster)  [unwired: 2 in, 1 out]
                n101 = property on="Zeitstempel 1 Ext" class="AbsZeit (strikt)"("Value"=w223) -> (error out=w220:errorcluster)  [unwired: 2 in, 1 out]
                n102 = property on="Zeitstempel" class="AbsZeit (strikt)"("Value"=w230) -> (error out=w227:errorcluster)  [unwired: 2 in, 1 out]
                n103 = property on="Zeitstempel 2" class="AbsZeit (strikt)"("Value"=w229) -> (error out=w226:errorcluster)  [unwired: 2 in, 1 out]
                n104 = Merge Errors(w220, w219, w218) -> (w212:errorcluster)
                n105 = Not(x=w246) -> (.not. x?=w245:bool)
                n106 = Index Array(array=w215, index=w217) -> (element=w209:string)
                n107 = Equal?(x="Warten", y=w209) -> (x = y?=w213:bool)
                n108 = call <vilib>:"Clear Errors.vi"("error in (no error)"=w212) -> ()  [unwired: 5 in, 2 out]
                n109 = Index Array(array=w216, index=w235) -> (element=w207:string)
                n110 = case shown="False" w240 {
                  tunnel: [u32 16777222 u32 0] -> w241
                  tunnel: [u32 13816530 u32 56345] -> w242
                  frame False {
                  }
                  frame True {
                  }
                }
                n111 = case shown="False" w245 {
                  tunnel: [u32 0 u32 16777222] -> w253
                  tunnel: [u32 56345 u32 13816530] -> w252
                  frame False {
                  }
                  frame True {
                  }
                }
                n112 = Equal?(x="Warten", y=w207) -> (x = y?=w210:bool)
                n113 = Merge Errors(w227, w226, w225) -> (w224:errorcluster)
                n114 = call "Texte in VIs uebersetzen.vi"("Sprachliste"=w205, "String zum Übersetzen"=w207) -> ("String zum Übersetzen"=w206:string)  [unwired: 9 in, 4 out]
                n115 = call "Texte in VIs uebersetzen.vi"("Sprachliste"=w205, "String zum Übersetzen"=w209) -> ("String zum Übersetzen"=w208:string)  [unwired: 9 in, 4 out]
                n116 = case shown="True" w210 {
                  tunnel: w236 -> [w256 w269]
                  tunnel: [w260 w266] -> w233
                  tunnel: w206 -> [w254 w263]
                  frame True {
                    n117 = Divide(x=w256, y=60.0) -> (x/y=w257:dbl)
                    n118 = Number To Decimal String(number=w257) -> (decimal integer string=w261:string)  [unwired: 1 in]
                    n119 = call <vilib>:"Space Constant.vi"() -> ("String"=w259:string)
                    n120 = Concatenate Strings(w254, w259, "-" ("String"), w259, w261, w259, "min" ("String")) -> (w260:string)
                  }
                  frame False {
                    n121 = Number To Decimal String(number=w269) -> (decimal integer string=w267:string)  [unwired: 1 in]
                    n122 = call <vilib>:"Space Constant.vi"() -> ("String"=w265:string)
                    n123 = Concatenate Strings(w263, w265, "-" ("String"), w265, w267, w265, "sec" ("String")) -> (w266:string)
                  }
                }
                n124 = property on="Stickstoff Befüllzeit" class="DigWert (strikt)"("NumText.TextColor"=w253, "NumText.BGColor"=w252) -> (error out=w247:errorcluster)  [unwired: 2 in, 1 out]
                n125 = property on="Stickstoff Befüllzeit Ext" class="DigWert (strikt)"("NumText.TextColor"=w241, "NumText.BGColor"=w242) -> (error out=w243:errorcluster)  [unwired: 2 in, 1 out]
                n126 = case shown="True" w213 {
                  tunnel: [w270 w275] -> w232
                  tunnel: w231 -> [_ w274]
                  tunnel: w208 -> [w270 w271]
                  frame True {
                  }
                  frame False {
                    n127 = call <vilib>:"Space Constant.vi"() -> ("String"=w273:string)
                    n128 = Concatenate Strings(w271, w273, "-" ("String"), w273, w274, w273, "sec" ("String")) -> (w275:string)
                  }
                }
                n129 = call <vilib>:"Clear Errors.vi"("error in (no error)"=w224) -> ()  [unwired: 5 in, 2 out]
                n130 = call <vilib>:"Clear Errors.vi"("error in (no error)"=w247) -> ()  [unwired: 5 in, 2 out]
                n131 = call <vilib>:"Clear Errors.vi"("error in (no error)"=w243) -> ()  [unwired: 5 in, 2 out]
              }
            }
            n132 = Unbundle By Name(w181) -> ("I6: Reserve"=w178:bool, "I0: N2 Nachf. FT-IR voll"=w174:bool, "I1: N2 Nachf. Vorrat leer"=w175:bool, "I9: Reserve"=w176:bool, "I10: Reserve"=w177:bool)
            n133 = case shown="True" w178 {
              tunnel: ["Externe Befüllung nicht vorhanden" w201] -> w193
              tunnel: w184 -> [_ w201]
              frame False {
              }
              frame True {
              }
            }
            n134 = Unbundle By Name(w170) -> ("O47: Statusbeleuchtung rot"=w169:bool)
            n135 = Unbundle By Name(w173) -> ("O16: N2 Einblasung"=w172:bool, "O17: LSP LN2 Nachfüllung"=w171:bool)
            n136 = Equal?(x="Warten", y=w186) -> (x = y?=w190:bool)
            n137 = Equal?(x="Befüllen", y=w186) -> (x = y?=w188:bool)
            n138 = Or(x=w190, y=w188) -> (x .or. y?=w191:bool)
            n139 = property on="Befüllung aktiv" class="Ring (strikt)"() -> (error out=w182:errorcluster, "Value"=w183:u16)  [unwired: 2 in, 1 out]
            n140 = local read "LN2 Cluster mit Ext"() -> (w179:T9)
            n141 = call <vilib>:"Clear Errors.vi"("error in (no error)"=w182) -> ()  [unwired: 5 in, 2 out]
            n142 = case shown="False" w191 {
              tunnel: [_ w202] -> w192
              tunnel: w185 -> [_ w202]
              frame False {
              }
              frame True {
              }
            }
            n143 = property on="Befüllung Extern aktiv" class="Ring (strikt)"() -> ("Value"=w180:u16)  [unwired: 2 in, 2 out]
            n144 = case shown="1" w183 {
              tunnel: ["Inaktiv!" w199] -> w164
              tunnel: w192 -> [_ w199]
              frame 0, Default {
              }
              frame 1 {
              }
            }
            n145 = case shown="0, Standard" w180 {
              tunnel: ["Inaktiv!" w197] -> w165
              tunnel: w193 -> [_ w197]
              frame 0, Default {
              }
              frame 1 {
              }
            }
            n146 = Bundle By Name(cluster=w179, "LS -17B3"=w177, "LS -16B2"=w175, "LS -17B2"=w176, "LS -16B1"=w174, "-16B7"=w178, "-22Y1"=w172, "-22Y2"=w171, "-22Y3"=w169) -> (w168:T9)
            n147 = call "Texte in VIs uebersetzen.vi"("Sprachliste"=w163, "String zum Übersetzen"=w164) -> ("String zum Übersetzen"=w161:string)  [unwired: 9 in, 4 out]
            n148 = call "Texte in VIs uebersetzen.vi"("Sprachliste"=w163, "String zum Übersetzen"=w165) -> ("String zum Übersetzen"=w160:string)  [unwired: 9 in, 4 out]
            n149 = property on="Status LN2 Befüllung" class="Str (strikt)"("Value"=w161) -> ()  [unwired: 2 in, 2 out]
            n150 = property on="Status LN2 Befüllung Ext." class="Str (strikt)"("Value"=w160) -> ()  [unwired: 2 in, 2 out]
            n151 = local write "LN2 Cluster mit Ext"(w168) -> ()
          }
        }
        n152 = Unbundle By Name(w123) -> ("FT-IR Kühlung Max"=w120:sgl)
        n153 = Unbundle By Name(w125) -> ("Rohwert Durchfluss FT-IR"=→"Rohwert FT-IR":sgl, "Rohwert Druck Ausgang"=→"Rohwert Ausgang":sgl, "Rohwert Druck FT-IR"=→"Rohwert Druck FT-IR":sgl, "AI3: Druck FT-IR"=→"FT-IR Druck Ist":sgl, "AI1: Druck Ausgang"=→"Druck Ausgang:":sgl, "AI2: Umgebungsdruck"=→"Druck Umgebung:":sgl, "Rohwert Umgebungsdruck"=→"Rohwert Umgebung":sgl)  [unwired: 1 out]
        n154 = control-ref of="FT-IR Kühlung Ist"() -> (w124:refnum<vi>)
        n155 = Unbundle By Name(w108) -> ("TC8: FT-IR"=→"FT-IR Kühlung Ist":sgl)
        n156 = call "Istwert Ueberwachung.vi"("Max"=w120, "Referernz"=w124) -> ()  [unwired: 10 in]
        n157 = call "FGV cRIO-Daten.vi"("Aktion"=enum16{"lesen", "schreiben"}."lesen") -> ("Analog Input"=w90:T28)  [unwired: 9 in, 9 out]
        n158 = Unbundle By Name(w90) -> ("AI0: Durchfluss FT-IR"=→"Durchfluss FTIR":sgl, "AI1: Druck Ausgang"=→"Druck Ausgang":sgl, "AI2: Umgebungsdruck"=→"Druck Umgebung":sgl, "AI3: Druck FT-IR"=→"Druck FTIR IAG":sgl, "AI4: Druck CalGas"=→"Druck CG":sgl, "Rohwert Durchfluss FT-IR"=→"Roh Durchfl.FTIR":sgl, "Rohwert Druck Ausgang"=→"Roh Druck Ausgang":sgl, "Rohwert Umgebungsdruck"=→"Roh Durck Umgebung":sgl, "Rohwert Druck FT-IR"=→"Roh Durck FTIR IAG":sgl, "Rohwert Druck CalGas"=→"Roh Durck CG":sgl)
        n159 = local read "Überwachung"() -> (w128:T8)
        n160 = Greater Than 0?(x=w128) -> (x > 0?=w127:bool)
        n161 = case shown="False" w127 {
          selector: w127 -> [w286 w287]
          tunnel: [u32 16777222 u32 16777222] -> w118
          tunnel: [w286 w287] -> w119
          frame False {
          }
          frame True {
          }
        }
        n162 = property on="Überwachung" class="Ring (strikt)"("Blinking"=w119, "RingText.TextColor"=w118) -> (error out=w112:errorcluster)  [unwired: 2 in, 1 out]
        n163 = call <vilib>:"Clear Errors.vi"("error in (no error)"=w112) -> ()  [unwired: 5 in, 2 out]
      }
      event "Manueller Betrieb": Value Change {
        n164 = event-data() -> ()  [unwired: 3 out]
        n165 = call "Gasringverdichter Test.vi"("Aktion"=enum16{"lesen", "Manuell B", "Speed"}."Manuell B", "Manueller Betrieb"="Manueller Betrieb") -> ()  [unwired: 8 in, 2 out]
      }
      event "Pumpendrehzahl": Value Change {
        n166 = event-data() -> ()  [unwired: 7 out]
        n167 = disable-structure shown="50l_N2_Tank==TRUE" {
          disable-tunnel: [w308 w314] -> w299
          disable-tunnel: [w307 w313] -> w298
          disable-tunnel: [w306 w312] -> w297
          disable-tunnel: ["LN2 normal" _] -> w296
          disable-tunnel: [_ w311] -> w295
          disable-tunnel: [_ w310] -> w294
          disable-tunnel: [_ "LN2 Cluster mit Ext"] -> w293
          frame condition #0 (active) {
            n168 = Unbundle By Name("LN2 normal") -> ("Befüllung aktiv"=w308:u16, "Stickstoff Befüllzeit"=w307:T5, "Befüllintervall"=w306:T5)
          }
          frame condition #1 {
            n169 = Unbundle By Name("LN2 Cluster mit Ext") -> ("Befüllung aktiv"=w314:u16, "Stickstoff Befüllzeit"=w313:T5, "Befüllintervall"=w312:T5, "Befüllung Extern aktiv"=w311:u16, "Stickstoff Befüllzeit Ext"=w310:T5)
          }
        }
        n170 = property on="speichern" class="Bool."("Visible"=TRUE ("Sichtbar")) -> (error out=w300:errorcluster)  [unwired: 2 in, 1 out]
        n171 = call "FGV Passwortlevel.vi"("FGV Passwort Aktion"=FGV_Passwort_Aktion."prüfen", "geforderter Level"=i16 8) -> ("Freigabe"=w301:bool)  [unwired: 2 in, 7 out]
        n172 = call <vilib>:"Clear Errors.vi"("error in (no error)"=w300) -> ()  [unwired: 5 in, 2 out]
        n173 = case shown="True" w301 {
          tunnel: w299 -> [_ w350]
          tunnel: w298 -> [_ w349]
          tunnel: w297 -> [_ w348]
          tunnel: w296 -> [w321 _]
          tunnel: w295 -> [_ w347]
          tunnel: w294 -> [_ w346]
          tunnel: w293 -> [w317 _]
          frame False {
            n174 = call "FGV Erweiterte Konfig.vi"("Aktion"=FGV_PID_Aktionen."Lesen") -> ("Sonstige"=w326:T20)  [unwired: 5 in, 5 out]
            n175 = Unbundle By Name(w326) -> ("Lüfter langsam"=w327:sgl, "Lüfter schnell"=w328:sgl, "FT-IR Kühlung Soll"=w329:sgl, "FT-IR Kühlung Max"=w330:sgl, "Überwachung"=w331:T8, "Befüllung aktiv"=w320:T19, "Befüllintervall"=w319:sgl, "Stickstoff Befüllzeit"=w318:sgl, "Kalibrierwert FT-IR"=w332:sgl, "Offset Ausgang"=w333:sgl, "Offset FT-IR"=w324:sgl, "Offset Druck FT-IR"=w323:sgl, "Offset Umgebung"=w322:sgl, "ext. Befüllung"=w316:T19, "Ext. Stickstoff Befüllzeit"=w315:sgl)
            n176 = local write "FT-IR Kühlung Max"(w330) -> ()
            n177 = local write "Lüfter langsam"(w327) -> ()
            n178 = local write "Überwachung"(w331) -> ()
            n179 = local write "Offset Ausgang"(w333) -> ()
            n180 = local write "Offset Druck FT-IR"(w323) -> ()
            n181 = local write "Offset Umgebung"(w322) -> ()
            n182 = local write "Kalib.FT-IR"(w332) -> ()
            n183 = local write "Schnell ab:"(w328) -> ()
            n184 = local write "Offset FT-IR"(w324) -> ()
            n185 = local write "°C"(w329) -> ()
            n186 = disable-structure shown="50l_N2_Tank==FALSE, Standard" {
              disable-tunnel: w321 -> [w338 _]
              disable-tunnel: w320 -> [w337 w343]
              disable-tunnel: w319 -> [w335 w342]
              disable-tunnel: w318 -> [w334 w341]
              disable-tunnel: w317 -> [_ w345]
              disable-tunnel: w316 -> [_ w340]
              disable-tunnel: w315 -> [_ w339]
              frame condition #0 (active) {
                n187 = Bundle By Name(cluster=w338, "Befüllung aktiv"=w337, "Befüllintervall"=w335, "Stickstoff Befüllzeit"=w334) -> (w336:T12)
                n188 = local write "LN2 normal"(w336) -> ()
              }
              frame condition #1 {
                n189 = Bundle By Name(cluster=w345, "Befüllung aktiv"=w343, "Befüllintervall"=w342, "Stickstoff Befüllzeit"=w341, "Befüllung Extern aktiv"=w340, "Stickstoff Befüllzeit Ext"=w339) -> (w344:T9)
                n190 = local write "LN2 Cluster mit Ext"(w344) -> ()
              }
            }
          }
          frame True {
            n191 = Bundle("Lüfter langsam"="Lüfter langsam", "Schnell ab:"="Schnell ab:", "°C"="°C", "FT-IR Kühlung Max"="FT-IR Kühlung Max", "Überwachung"="Überwachung", "Befüllung aktiv"=w350, "Stickstoff Befüllzeit"=w349, "Befüllintervall"=w348, "Kalib.FT-IR"="Kalib.FT-IR", "Offset Ausgang"="Offset Ausgang", "Offset FT-IR"="Offset FT-IR", "Offset Druck FT-IR"="Offset Druck FT-IR", "Dichtheitstest Zeit"="Dichtheitstest Zeit", "Dichtheitstest Abfall"="Dichtheitstest Abfall", "Dichtheitstest Umfang"="Dichtheitstest Umfang", "Offset Umgebung"="Offset Umgebung", "Max Taupunkt"="Max Taupunkt", "Pumpendrehzahl"="Pumpendrehzahl", "Befüllung Extern aktiv"=w347, "Stickstoff Befüllzeit Ext"=w346) -> (w362:T30)  [unwired: 1 in]
            n192 = call "FGV Erweiterte Konfig.vi"("Aktion"=FGV_PID_Aktionen."Schreiben Sonstige", "Sonstige"=w362) -> ()  [unwired: 4 in, 6 out]
          }
        }
      }
      event Value Change {
        n193 = event-data() -> ()  [unwired: 2 out]
        n194 = vi-ref "T90.lvlib:T90 konfig.vi"() -> (w369:refnum<vi>)
        n195 = call "VI Pop Up.vi"("VI Referenz"=w369) -> ()  [unwired: 10 in, 1 out]
      }
      event Value Change {
        n196 = event-data() -> ()  [unwired: 2 out]
        n197 = vi-ref "Erweiterte Konfig.lvlib:Parameter Druck Sensoren.vi"() -> (w371:refnum<vi>)
        n198 = call "VI Pop Up.vi"("VI Referenz"=w371) -> ()  [unwired: 10 in, 1 out]
      }
      event Value Change {
        n199 = event-data() -> ()  [unwired: 2 out]
        n200 = call "FGV Passwortlevel.vi"("FGV Passwort Aktion"=FGV_Passwort_Aktion."prüfen", "geforderter Level"=i16 8) -> ("Freigabe"=w374:bool)  [unwired: 2 in, 7 out]
        n201 = case shown="True" w374 {
          frame False {
          }
          frame True {
            n202 = vi-ref "Erweiterte Konfig.lvlib:PID-Parameter Druckregler einstellen v2.vi"() -> (w376:refnum<vi>)
            n203 = call "VI Pop Up.vi"("VI Referenz"=w376) -> ()  [unwired: 10 in, 1 out]
          }
        }
        n204 = disable-structure shown="Deaktiviert" {
          frame Disabled {
            n205 = call "PID-Parameter Druckregler.vi"() -> ()  [unwired: 12 in]
          }
          frame Enabled {
          }
        }
      }
      event Value Change {
        n206 = event-data() -> ("NewVal"=w378:T14, "OldVal"=w381:T14)  [unwired: 1 out]
        n207 = call "FGV Passwortlevel.vi"("FGV Passwort Aktion"=FGV_Passwort_Aktion."prüfen", "geforderter Level"=i16 8) -> ("Freigabe"=w383:bool)  [unwired: 2 in, 7 out]
        n208 = property on="speichern" class="Bool."("Visible"=TRUE ("Sichtbar")) -> (error out=w379:errorcluster)  [unwired: 2 in, 1 out]
        n209 = case shown="True" w383 {
          tunnel: w378 -> [_ w386]
          tunnel: w381 -> [w385 _]
          frame False {
            n210 = local write "PID-Parameter Anzeige"(w385) -> ()
          }
          frame True {
            n211 = call "FGV Erweiterte Konfig.vi"("Aktion"=FGV_PID_Aktionen."Schreiben PID", "PID-Parameter Anzeige"=w386) -> ()  [unwired: 4 in, 6 out]
          }
        }
        n212 = call <vilib>:"Clear Errors.vi"("error in (no error)"=w379) -> ()  [unwired: 5 in, 2 out]
      }
      event Value Change {
        n213 = event-data() -> ()  [unwired: 2 out]
        n214 = flat-sequence {
          frame #0 {
            n215 = call "Daten am cRIO Speichern.vi"("Aktionen"=Aktionen_Daten_am_cRIO_speichern."speichern setzen") -> ()  [unwired: 9 in, 2 out]
          }
          frame #1 {
            n216 = vi-ref "Bitte Warten.vi"() -> (w390:refnum<vi>)
            n217 = call "VI Pop Up.vi"("VI Referenz"=w390) -> ()  [unwired: 10 in, 1 out]
          }
          frame #2 {
            n218 = property on="speichern" class="Bool."("Visible"=FALSE ("Sichtbar")) -> (error out=w391:errorcluster)  [unwired: 2 in, 1 out]
            n219 = call <vilib>:"Clear Errors.vi"("error in (no error)"=w391) -> ()  [unwired: 5 in, 2 out]
          }
        }
      }
      event Value Change {
        n220 = event-data() -> ()  [unwired: 2 out]
        n221 = call "FGV Passwortlevel.vi"("FGV Passwort Aktion"=FGV_Passwort_Aktion."prüfen", "geforderter Level"=i16 5) -> ("Freigabe"=w394:bool)  [unwired: 2 in, 7 out]
        n222 = case shown="True" w394 {
          frame False {
          }
          frame True {
            n223 = vi-ref "AK-Schnittstelle.lvlib:Konfig AK.vi"() -> (w397:refnum<vi>)
            n224 = call "VI Pop Up.vi"("VI Referenz"=w397) -> ()  [unwired: 10 in, 1 out]
          }
        }
      }
      event Value Change {
        n225 = event-data() -> ()  [unwired: 2 out]
        n226 = vi-ref "Status Steuerung.vi"() -> (w399:refnum<vi>)
        n227 = call "VI Pop Up.vi"("VI Referenz"=w399) -> ()  [unwired: 10 in, 1 out]
      }
      event Value Change {
        n228 = event-data() -> ()  [unwired: 2 out]
        n229 = flat-sequence {
          frame #0 {
            n230 = call "FGV Erweiterte Konfig.vi"("Aktion"=FGV_PID_Aktionen."Dichtheitstest", "Dichtheitstest?"=TRUE) -> ()  [unwired: 5 in, 5 out]
            n231 = call "FGV-Funktionstasten.vi"("Zustand"=Zustaende."Standby", "Aktion"=Funktionstasten-Aktion."Zustand setzen") -> ()  [unwired: 6 in, 8 out]
          }
          frame #1 {
            n232 = vi-ref "Dichtheitstest.vi"() -> (w405:refnum<vi>)
            n233 = call "VI Pop Up.vi"("VI Referenz"=w405) -> ()  [unwired: 10 in, 1 out]
          }
        }
      }
      event Value Change {
        n234 = event-data() -> ()  [unwired: 7 out]
        n235 = vi-ref "O2 Dichtheitstest.lvlib:O2 main.vi"() -> (w407:refnum<vi>)
        n236 = call "VI Pop Up.vi"("VI Referenz"=w407) -> ()  [unwired: 10 in, 1 out]
      }
      event Value Change {
        n237 = event-data() -> ()  [unwired: 2 out]
        n238 = vi-ref "Erweiterte Konfig.lvlib:CG-Check Konfig.lvlib:VI CG-Check Konfig.vi"() -> (w409:refnum<vi>)
        n239 = call "VI Pop Up.vi"("VI Referenz"=w409) -> ()  [unwired: 10 in, 1 out]
      }
      event Value Change {
        n240 = event-data() -> ("OldVal"=w412:T13)  [unwired: 1 out]
        n241 = property on="speichern" class="Bool."("Visible"=TRUE ("Sichtbar")) -> (error out=w411:errorcluster)  [unwired: 2 in, 1 out]
        n242 = call <vilib>:"Clear Errors.vi"("error in (no error)"=w411) -> ()  [unwired: 5 in, 2 out]
        n243 = call "FGV Passwortlevel.vi"("FGV Passwort Aktion"=FGV_Passwort_Aktion."prüfen", "geforderter Level"=i16 8) -> ("Freigabe"=w416:bool)  [unwired: 7 in, 2 out]
        n244 = case shown="True" w416 {
          tunnel: "Parameter Sensoren" -> [_ w419]
          tunnel: w412 -> [w418 _]
          frame False {
            n245 = local write "Parameter Sensoren"(w418) -> ()
          }
          frame True {
            n246 = call "FGV Erweiterte Konfig.vi"("Aktion"=FGV_PID_Aktionen."Parameter Sensor", "Parameter Sensoren"=w419) -> ()  [unwired: 4 in, 6 out]
          }
        }
      }
    }
  }
  n247 = disable-structure shown="Deaktiviert" {
    frame Disabled {
      n248 = call "FGV Passwortlevel.vi"("FGV Passwort Aktion"=FGV_Passwort_Aktion."lesen") -> ("aktueller Level"=w422:i16)  [unwired: 8 in, 2 out]
      n249 = Greater Or Equal?(x=w422, y=i16 9) -> (x >= y?=w424:bool)
      n250 = property on="Gasringverdichter Speed" class="Drehknopf (strikt)"() -> (error out=w426:errorcluster, "Visible"=w425:bool)  [unwired: 2 in, 1 out]
      n251 = property on="Gasringverdichter Speed" class="Drehknopf (strikt)"("Visible"=w424) -> ()  [unwired: 2 in, 2 out]
      n252 = property on="Manueller Betrieb" class="Bool. (strikt)"("Visible"=w424) -> ()  [unwired: 2 in, 2 out]
      n253 = call <vilib>:"Clear Errors.vi"("error in (no error)"=w426) -> ()  [unwired: 5 in, 2 out]
      n254 = case shown="True" w425 {
        frame False {
        }
        frame True {
          n255 = Multiply(x="Gasringverdichter Speed", y=100.0) -> (x*y=w428:dbl)
          n256 = To Unsigned Word Integer(number=w428) -> (unsigned 16bit integer=w427:u16)
          n257 = call "Gasringverdichter Test.vi"("Aktion"=enum16{"lesen", "Manuell B", "Speed"}."Speed", "Speed"=w427) -> ()  [unwired: 8 in, 2 out]
        }
      }
    }
    frame Enabled {
    }
  }
  n258 = disable-structure shown="Deaktiviert" {
    frame Disabled {
      n259 = property on="PMA unsichtbar schalten" class="Bool. (strikt)"("Visible"=TRUE ("Sichtbar")) -> ()  [unwired: 2 in, 2 out]
    }
    frame Enabled {
    }
  }
